vi "PV Packet 1.vi"(11 "HEX Data (U8) in":u8[](array[numeric]) format="%x") -> (3 "PV Data 1":string[](array[string]))   [LabVIEW 2023]
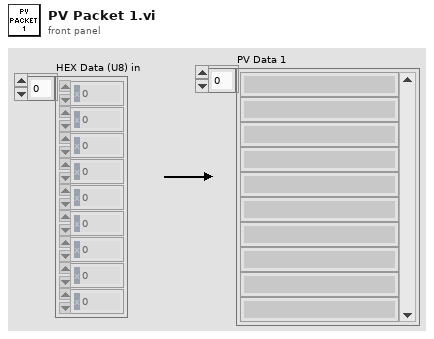
[diagram p1: front panel]
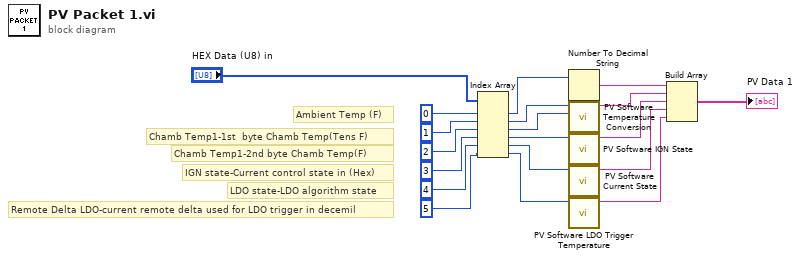
[diagram p0: block diagram]
diagram:
  # "Remote Delta LDO-current remote delta used for LDO trigger in decemil"
  # "LDO state-LDO algorithm state"
  # "IGN state-Current control state in (Hex)"
  # "Chamb Temp1-2nd byte Chamb Temp(F)"
  # "Chamb Temp1-1st  byte Chamb Temp(Tens F)"
  # "Ambient Temp (F)"
  n1 = Index Array(array="HEX Data (U8) in", index #1=0 ("disabled index (col)"), index #2=1 ("disabled index (col)"), index #3=2 ("disabled index (col)"), index #4=3 ("disabled index (col)"), index #5=4 ("disabled index (col)"), index #6=5 ("disabled index (col)")) -> (element #1=w8:u8, element #2=w9:u8, element #3=w10:u8, element #4=w11:u8, element #5=w13:u8, element #6=w12:u8)
  n2 = Number To Decimal String(number=w8) -> (decimal integer string=w14:string)  [unwired: 1 in]
  n3 = call "PV Software Temperature Conversion.vi"("HEX Data (Byte 2)"=w10, "HEX Data (Byte 1)"=w9) -> ("Temperature (F)"=w15:string)  [unwired: 9 in]
  n4 = call "PV Software IGN State.vi"("HEX Data (U8)"=w11) -> ("IGN State"=w16:string)  [unwired: 10 in]
  n5 = call "PV Software Current State.vi"("HEX Data (U8)"=w13) -> ("Current State"=w17:string)  [unwired: 10 in]
  n6 = call "PV Software LDO Trigger Temperature.vi"("HEX Data (U8)"=w12) -> ("LDO Trigger Temperature"=w18:string)  [unwired: 10 in]
  n7 = Build Array(w14, w15, w16, w17, w18) -> (→"PV Data 1":string[])
